vi "CustomPID_v4.0.vi"(0 "PID Tuning Parameters":T1={"Kp"=0.1, "Ki"=0.1, "Kd"=0.1, "N-Diff"=10, "N-Int"=20, "Int Error Window"=0.5, "Max Ouput"=1.0, "Min Output"=-1.0} {"Int Error Window" min=0.0; "N-Int" min=2; "N-Diff" min=2; "Kd" min=0.0; "Ki" min=0.0; "Kp" min=0.0}, 1 "Goal":dbl(slide) scale=-1.0..1.0, 2 "Process Variable":dbl(slide) scale=-1.0..1.0, 3 "Custom Error Calculation":dbl(slide) scale=-1.0..1.0, 7 "Reset on Goal Change ?":bool, 9 "Use Custom Error Calculation ?":bool, 12 "Reinit":bool) -> (4 "Command":dbl format="%_4g", 6 "Is Reset":bool, 8 "Current Error":dbl format="%_4g", 15 "Controller Summary":T2(graph))   [LabVIEW 2020]
doc: "Brief PID Description:\n\nA good mechanical analogy for a PID algorithm is a spring-mass system with a viscous damper \n(https://ccrma.stanford.edu/CCRMA/Courses/150/img35.gif). The proportional term is the \"spring,\" it has the strongest influence when the robot system is furthest from its goal. The derivative term is the damping coefficient, it's what allows the system to stop oscillating and reach it's goal. The integral term mostly comes into play if the robot has been been trying to move for a lengthy amount of time but still isn't able to reach it's goal (this is referred to as steady-state error).\n\nRecommended Tuning Procedure:\n\n1) You may want to restrict the Max and Min Output parameters more than [-1, 1] during initial tuning to avoid damaging the system.\n2) If you do not wish to pre-calculate a Kp, carefully increase the Kp term from 0.0001 until the system starts moving.\n3) If the system is going the wrong direction, you may need to negate the Command.\n4) Continue inceasing Kp until the system oscillates about the Goal.\n5) Carefully increase Kd from 0.0001 until the system's response is sufficiently damped (i.e. until the oscillation is mitigated).\n6) Carefully increase Ki from 0.0001 to reduce the steady-state error (SSE) (if any).\n7) Adjust N-Diff if necessary (minimum of 2). Increasing N-Diff will reduce the effects of sensor (Process Variable) noise on the \nderivative term but will increase the lag on that component. You may also want to add a filter to Process Variable data.\n8) Adjust N-Int if necessary (minimum of 2). Increasing N-Int may help the system overcome SSE but may also increase integrator wind-up. It will also increase the lag for that component.\n9) Another way to reduce integrator wind-up is to set the Integral Error Window. The Intergral term will only be used if the magnitude of the error is less than the specified window.\n10) You may need to adjust Ki, and Kd after adjusting N-Diff and N-Int, respectively. \n\nAdditional Notes:\n\n1) Make sure that execution type for all instances of this VI are set to \"preallocated clone reentrant execution.\"\n2) Several parts of this VI were inspired by a PID algorithm written by Dr. Ira Hill at the University of Florida and have been developed in collaboration with FRC 2614.\n3) If you have any questions, feel free to contact me at lrscime.alpha@gmail.coms"
uses:
  <vilib>/Analysis/6fits.llb/Curve Fitting Criteria.ctl
  <vilib>/Analysis/NI_AALPro.lvlib
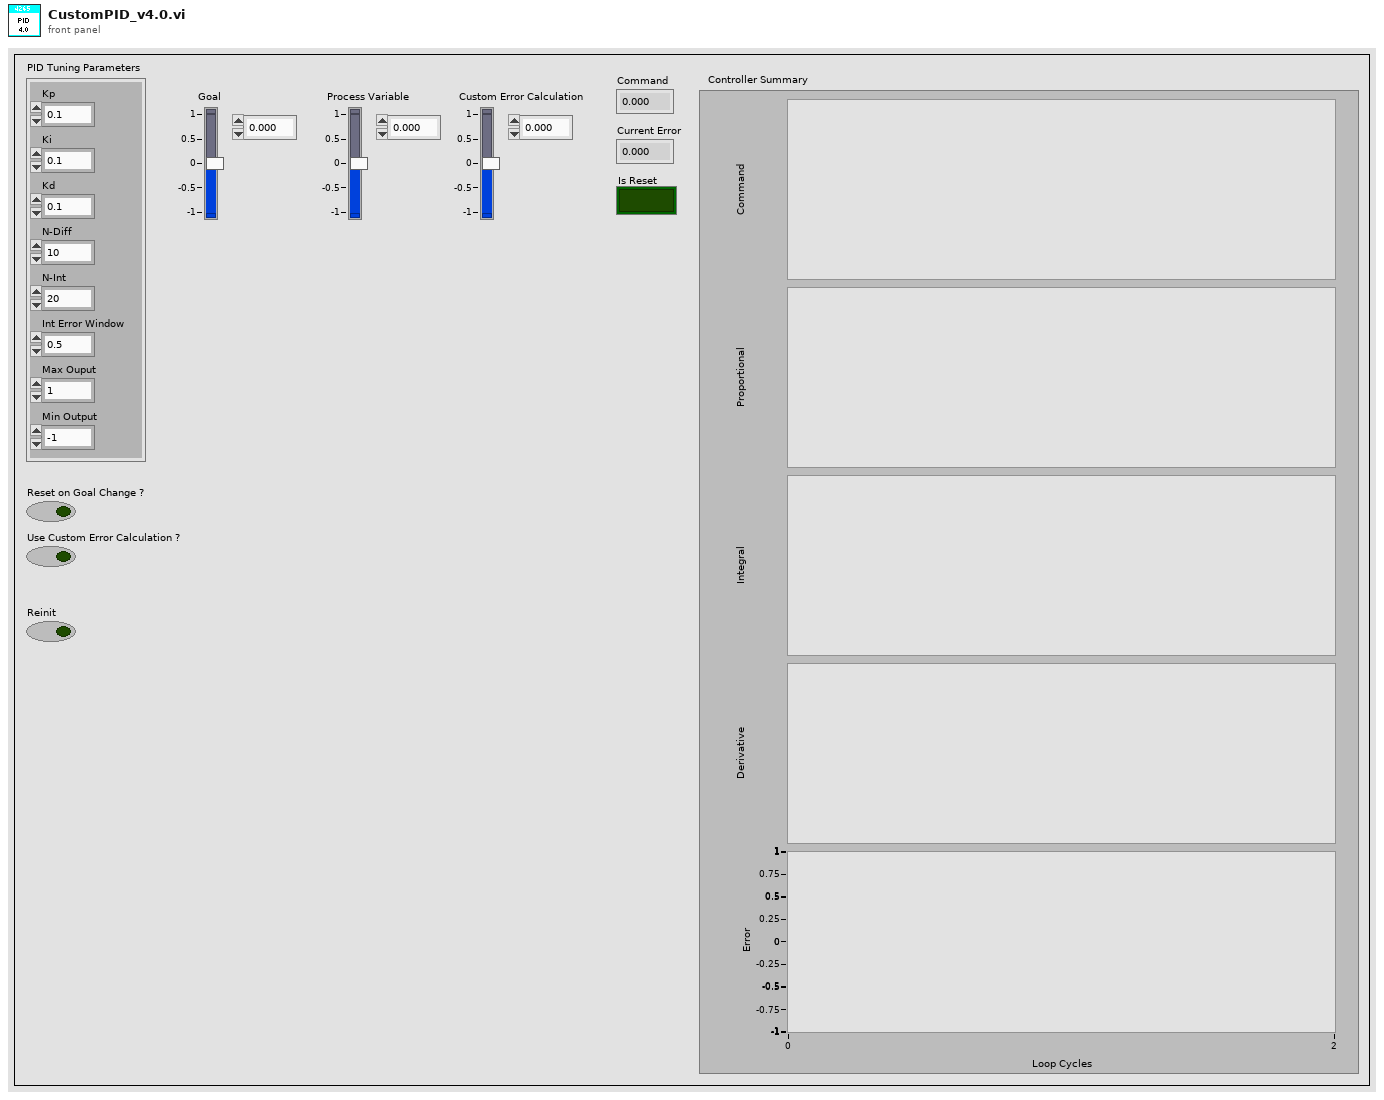
[diagram p1: front panel]
types:
  T1 = cluster{"Kp":dbl, "Ki":dbl, "Kd":dbl, "N-Diff":i32, "N-Int":i32, "Int Error Window":dbl, "Max Ouput":dbl, "Min Output":dbl}
  T2 = cluster{"Command":dbl, "Proportional":dbl, "Integral":dbl, "Derivative":dbl, "Goal":dbl}
  T3 = cluster{"Command":dbl, "Proportional":dbl, "Integral":dbl, "Derivative":dbl, "Error":dbl}
  T4 = typedef "NI_AALPro.lvlib/Curve Fitting Criteria.ctl" = u16
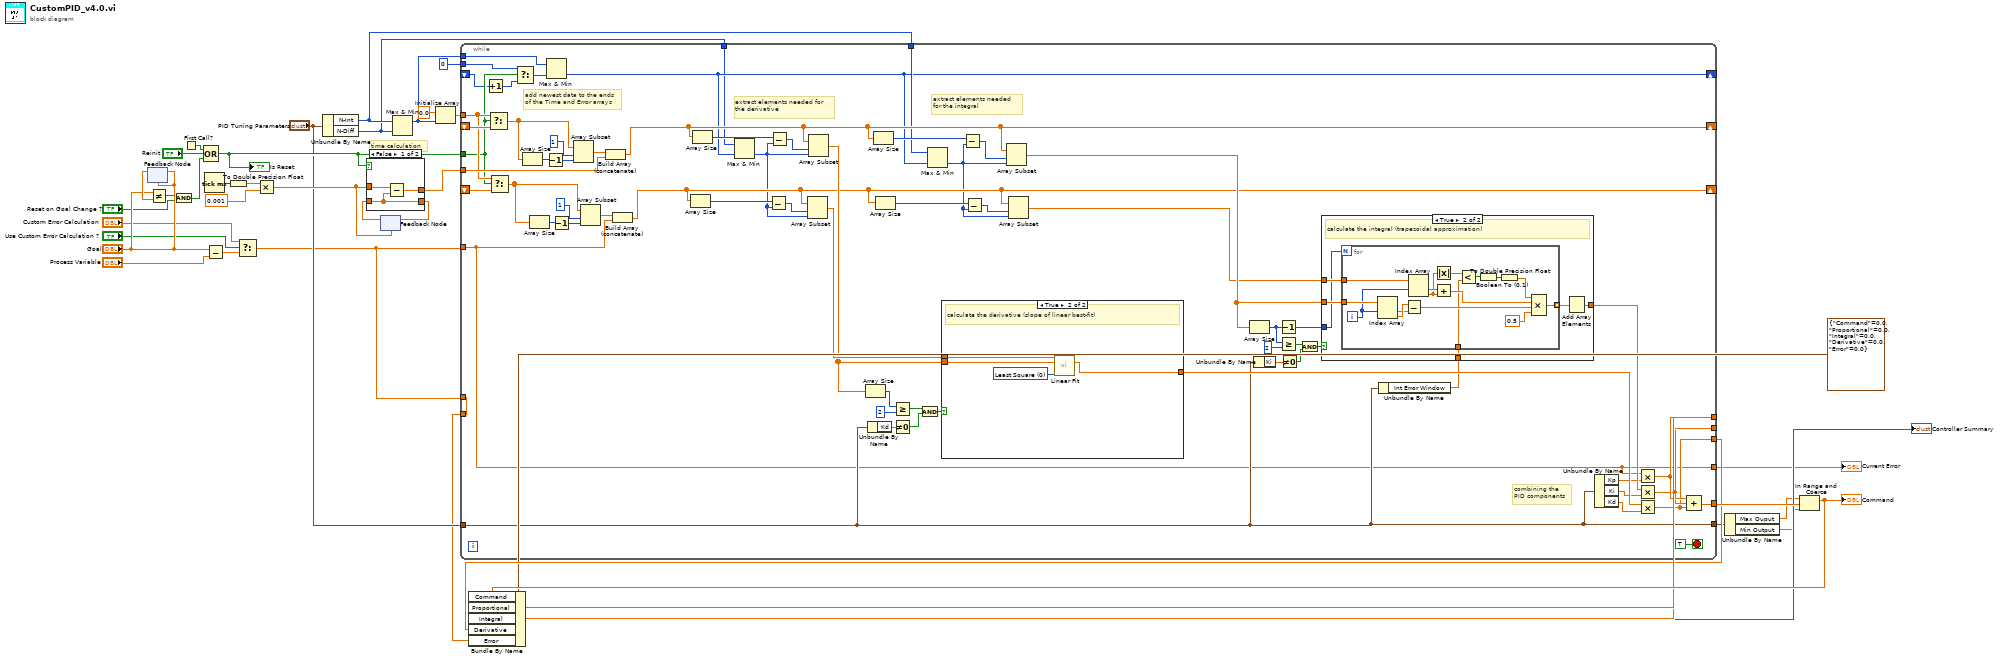
[diagram p0: block diagram]
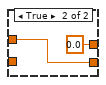
[diagram p2: hidden frame]
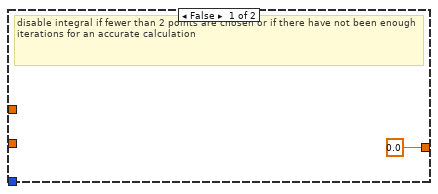
[diagram p3: hidden frame]
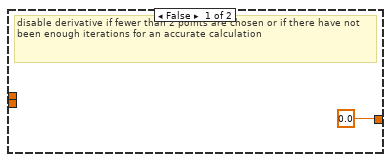
[diagram p4: hidden frame]
diagram:
  # "time calculation"
  n1 = feedback #1("Goal") -> (w34:dbl)
  n2 = feedback-in #1("Goal") -> ()
  n3 = Not Equal?(x="Goal", y=w34) -> (x != y?=w17:bool)
  n4 = And(x=w17, y="Reset on Goal Change ?") -> (x .and. y?=w27:bool)
  n5 = First Call?() -> (First Call?: T/F=w38:bool)
  n6 = Compound Arithmetic op=OR(w38, "Reinit", w27) -> (w28:bool)
  "Is Reset" <- w28
  n7 = Tick Count (ms)() -> (millisecond timer value=w33:u32)
  n8 = Subtract(x="Goal", y="Process Variable") -> (x-y=w15:dbl)
  n9 = To Double Precision Float(number=w33) -> (double precision float=w32:dbl)
  n10 = Select(t="Custom Error Calculation", s="Use Custom Error Calculation ?", f=w15) -> (s? t:f=w1:dbl)
  n11 = Multiply(x=w32, y=0.001) -> (x*y=w26:dbl)
  n12 = Unbundle By Name("PID Tuning Parameters") -> ("N-Int"=w10:i32, "N-Diff"=w9:i32)
  n13 = feedback #2(w26) -> (w29:dbl)
  n14 = case shown="False" w28 {
    tunnel: w26 -> [w42 w44]
    tunnel: [w40 w44] -> w30
    tunnel: [w41 0.0] -> w20
    tunnel: w29 -> [w40 _]
    frame False {
      n15 = Subtract(x=w42, y=w40) -> (x-y=w41:dbl)
    }
    frame True {
    }
  }
  n16 = feedback-in #2(w30) -> ()
  n17 = Max & Min(x=w10, y=w9) -> (max(x,y)=w11:i32)  [unwired: 1 out]
  n18 = Initialize Array(0.0 ("element"), w11) -> (w36:dbl[])
  n19 = while {
    tunnel: [w109] -> w39
    tunnel: w1 -> [w46]
    shift-right: [w90] -> _
    shift-left: _ -> [w83]
    tunnel: w20 -> [w104]
    shift-right: [w84] -> _
    shift-left: _ -> [w80]
    tunnel: w28 -> [w71]
    tunnel: w36 -> [w81]
    tunnel: [w46] -> w13
    tunnel: [w76] -> w24
    tunnel: [w75] -> w23
    tunnel: [w74] -> w22
    tunnel: 0 -> [w72]
    shift-right: [w55] -> _
    shift-left: _ -> [w69]
    tunnel: w11 -> [w66]
    tunnel: w10 -> [w56]
    tunnel: w9 -> [w54]
    tunnel: "PID Tuning Parameters" -> [w47]
    tunnel: [w47] -> w7
    tunnel: [w45] -> w2
    tunnel: w1 -> [w45]
    stop <- TRUE stop-if-true
    # "combining the\nPID components"
    # "add newest data to the ends\nof the Time and Error arrays"
    # "extract elements needed for the integral"
    # "extract elements needed for the derivative"
    n20 = Increment(x=w69) -> (x+1=w70:i32)
    n21 = Select(t=w81, s=w71, f=w83) -> (s? t:f=w82:dbl[])
    n22 = Select(t=w81, s=w71, f=w80) -> (s? t:f=w79:dbl[])
    n23 = Select(t=w72, s=w71, f=w70) -> (s? t:f=w67:i32)
    n24 = Array Size(array=w82) -> (size(s)=w107:i32)
    n25 = Array Size(array=w79) -> (size(s)=w102:i32)
    n26 = Decrement(x=w107) -> (x-1=w106:i32)
    n27 = Max & Min(x=w66, y=w67) -> (min(x,y)=w55:i32)  [unwired: 1 out]
    n28 = Decrement(x=w102) -> (x-1=w101:i32)
    n29 = Array Subset(array=w82, index=1, length=w106) -> (w105:dbl[])
    n30 = Array Subset(array=w79, index=1, length=w101) -> (w100:dbl[])
    n31 = Build Array (concatenate)(w105, w104) -> (w90:dbl[])
    n32 = Build Array (concatenate)(w100, w46) -> (w84:dbl[])
    n33 = Array Size(array=w84) -> (size(s)=w96:i32)
    n34 = Array Size(array=w90) -> (size(s)=w99:i32)
    n35 = Max & Min(x=w54, y=w55) -> (min(x,y)=w68:i32)  [unwired: 1 out]
    n36 = Subtract(x=w96, y=w68) -> (x-y=w97:i32)
    n37 = Subtract(x=w99, y=w68) -> (x-y=w98:i32)
    n38 = Array Subset(array=w84, index=w97, length=w68) -> (w95:dbl[])
    n39 = Array Subset(array=w90, index=w98, length=w68) -> (w94:dbl[])
    n40 = Array Size(array=w94) -> (size(s)=w73:i32)
    n41 = Unbundle By Name(w47) -> ("Kd"=w53:dbl)
    n42 = Array Size(array=w90) -> (size(s)=w92:i32)
    n43 = Array Size(array=w84) -> (size(s)=w89:i32)
    n44 = Greater Or Equal?(x=w73, y=2) -> (x >= y?=w65:bool)
    n45 = Not Equal To 0?(x=w53) -> (x != 0?=w63:bool)
    n46 = Compound Arithmetic op=AND(w65, w63) -> (w64:bool)
    n47 = Max & Min(x=w56, y=w55) -> (min(x,y)=w62:i32)  [unwired: 1 out]
    n48 = case shown="True" w64 {
      tunnel: w95 -> [_ w138]
      tunnel: w94 -> [_ w137]
      tunnel: [0.0 w135] -> w77
      frame False {
        # "disable derivative if fewer than 2 points are chosen or if there have not been enough iterations for an accurate calculation"
      }
      frame True {
        w136 = T4 0 items=["Least Square", "Least Absolute Residual", "Bisquare"] ("method")
        # "calculate the derivative (slope of linear best-fit)"
        n49 = call <vilib>:"Linear Fit.vi"("Y"=w138, "X"=w137, "method"=w136) -> ("slope"=w135:dbl)  [unwired: 8 in, 4 out]
      }
    }
    n50 = Subtract(x=w92, y=w62) -> (x-y=w91:i32)
    n51 = Subtract(x=w89, y=w62) -> (x-y=w88:i32)
    n52 = Array Subset(array=w90, index=w91, length=w62) -> (w85:dbl[])
    n53 = Array Subset(array=w84, index=w88, length=w62) -> (w78:dbl[])
    n54 = Array Size(array=w85) -> (size(s)=w61:i32)
    n55 = Unbundle By Name(w47) -> ("Ki"=w52:dbl)
    n56 = Decrement(x=w61) -> (x-1=w60:i32)
    n57 = Greater Or Equal?(x=w61, y=2) -> (x >= y?=w59:bool)
    n58 = Not Equal To 0?(x=w52) -> (x != 0?=w57:bool)
    n59 = Compound Arithmetic op=AND(w59, w57) -> (w58:bool)
    n60 = Unbundle By Name(w47) -> ("Int Error Window"=w51:dbl)
    n61 = case shown="True" w58 {
      tunnel: [0.0 w112] -> w86
      tunnel: w85 -> [_ w117]
      tunnel: w78 -> [_ w116]
      tunnel: w51 -> [_ w115]
      tunnel: w60 -> [_ w114]
      frame False {
        # "disable integral if fewer than 2 points are chosen or if there have not been enough iterations for an accurate calculation"
      }
      frame True {
        # "calculate the integral (trapezoidal approximation)"
        n62 = for {
          N: w114 -> [_]
          tunnel: w117 -> [w133]
          tunnel: w116 -> [w127]
          tunnel: w115 -> [w120]
          tunnel: [w119] -> w113 mode=indexing
          i -> [w128]
          n63 = Index Array(array=w133, index #1=w128) -> (element #1=w131:dbl, element #2=w132:dbl)  [unwired: 1 in]
          n64 = Subtract(x=w132, y=w131) -> (x-y=w130:dbl)
          n65 = Index Array(array=w127, index #1=w128) -> (element #1=w125:dbl, element #2=w118:dbl)  [unwired: 1 in]
          n66 = Absolute Value(x=w118) -> (abs(x)=w124:dbl)
          n67 = Add(x=w125, y=w118) -> (x+y=w126:dbl)
          n68 = Less?(x=w124, y=w120) -> (x < y?=w123:bool)
          n69 = Boolean To (0,1)(Boolean=w123) -> (0, 1=w122:i16)
          n70 = To Double Precision Float(number=w122) -> (double precision float=w121:dbl)
          n71 = Compound Arithmetic op=MULTIPLY(w121, w126, w130, 0.5 ("value")) -> (w119:dbl)
        }
        n72 = Add Array Elements(numeric array=w113) -> (sum=w112:dbl)
      }
    }
    n73 = Unbundle By Name(w47) -> ("Kp"=w50:dbl, "Ki"=w49:dbl, "Kd"=w48:dbl)
    n74 = Multiply(x=w46, y=w50) -> (x*y=w76:dbl)
    n75 = Multiply(x=w86, y=w49) -> (x*y=w75:dbl)
    n76 = Multiply(x=w77, y=w48) -> (x*y=w74:dbl)
    n77 = Compound Arithmetic op=ADD(w76, w75, w74) -> (w109:dbl)
  }
  "Current Error" <- w13
  n78 = Unbundle By Name(w7) -> ("Max Ouput"=w6:dbl, "Min Output"=w5:dbl)
  n79 = In Range and Coerce(upper limit=w6, x=w39, lower limit=w5) -> (coerced(x)=w25:dbl)  [unwired: 1 out]
  "Command" <- w25
  n80 = Bundle By Name(cluster=T3 {"Command"=0.0, "Proportional"=0.0, "Integral"=0.0, "Derivative"=0.0, "Error"=0.0} ("input cluster"), "Command"=w25, "Proportional"=w24, "Integral"=w23, "Derivative"=w22, "Error"=w2) -> (→"Controller Summary":T3)
